vi "Run Scripting in Project Context.vi"(6 "Scripting VI":refnum<vi>, 11 "Project":refnum<vi>) -> (0 "error out":errorcluster)   [LabVIEW 2020]
doc: "Runs the specified project scripting VI in the context of the project. This avoids any issues with classes getting opened in a persistent tools menu context and keeping classes locked."
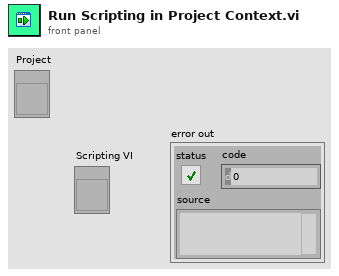
[diagram p1: front panel]
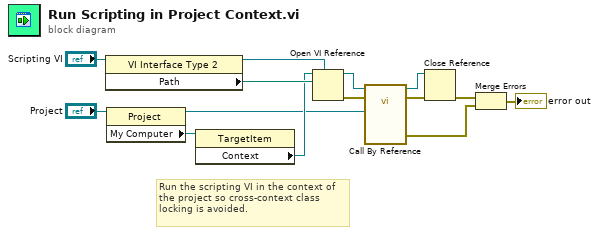
[diagram p0: block diagram]
diagram:
  # "Run the scripting VI in the context of the project so cross-context class locking is avoided."
  n1 = property class="VI Interface Type 2"(reference="Scripting VI") -> (reference out=w12:refnum<vi>, "Path"=w13:path)  [unwired: 1 in, 1 out]
  n2 = property class="Project"(reference="Project") -> (reference out=w6:refnum<vi>, "My Computer"=w10:refnum<vi>)  [unwired: 1 in, 1 out]
  n3 = property class="TargetItem"(reference=w10) -> ("Context"=w9:refnum<vi>)  [unwired: 1 in, 2 out]
  n4 = Open VI Reference(type specifier VI Refnum (for type only)=w12, application reference (local)=w9, vi path=w13) -> (vi reference=w7:refnum<vi>, error out=w8:errorcluster)  [unwired: 3 in]
  n5 = call-by-ref "?"(reference=w7, error in=w8, "Project"=w6) -> (reference out=w4:refnum<vi>, error out=w5:errorcluster, 0:"error out"=w2:errorcluster)  [unwired: 10 in]
  n6 = Close Reference(reference=w4, error in (no error)=w5) -> (error out=w3:errorcluster)
  n7 = Merge Errors(w3, w2) -> (→"error out":errorcluster)
